vi "Generate Non Text Layer(s).vi"(0 "Library Path":path, 5 "new picture":picture, 11 "error in":errorcluster) -> (4 "Layers":refnum<class "Layer.lvclass">[](array[class]), 15 "error out":errorcluster)   [LabVIEW 2020, in "Text-Based VI Icon.lvlib"]
uses:
  <vilib>/LabVIEW Icon API/Set Text Icon/Text-Based VI Icon.lvlib
  <vilib>/LabVIEW Icon API/lv_icon/Classes/Layer/Layer.lvclass
  <vilib>/LabVIEW Icon API/lv_icon/Controls/Layer.ctl
  <vilib>/LabVIEW Icon API/Set Text Icon/User Visible Strings.vi
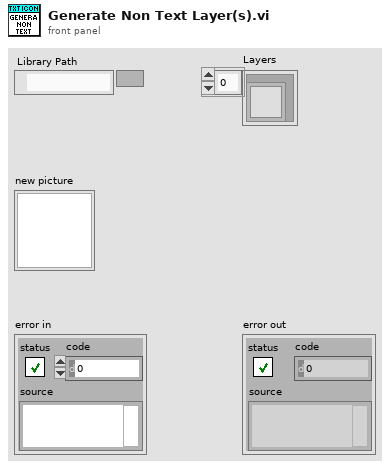
[diagram p1: front panel]
types:
  T1 = cluster{"left":i16, "top":i16, "right":i16, "bottom":i16}
  T2 = typedef "Layer.ctl" = cluster{"LayerIcon":picture, "LayerName":string, "Opacity":u8, "Visibility?":bool}
  T3 = typedef "imagedata.ctl" = cluster{"image type":i32, "image depth":i32, "image":u8[], "mask":u8[], "colors":u32[], "Rectangle":cluster{"left":i16, "top":i16, "right":i16, "bottom":i16}}
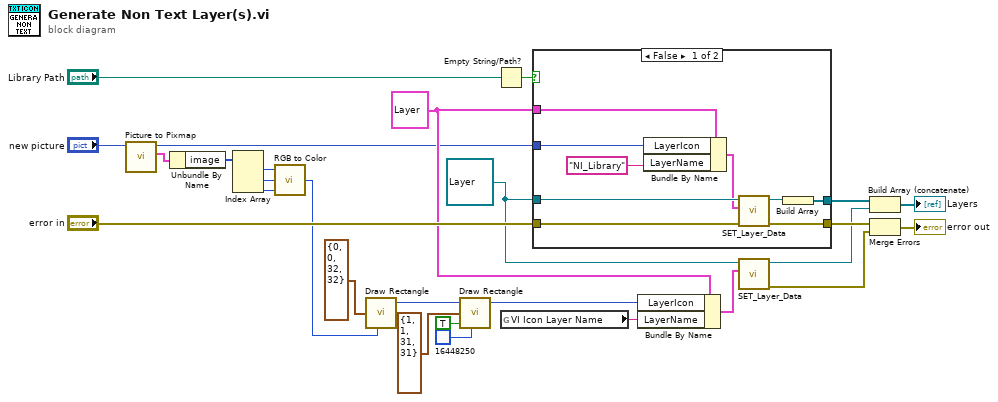
[diagram p0: block diagram]
diagram:
  w9 = T2 {"LayerIcon"=bytes[3102], "LayerName"="", "Opacity"=100, "Visibility?"=TRUE} ("Data")
  w25 = refnum<class "Layer.lvclass"> refnum ("Layer.lvclass in")
  n1 = call <vilib>:"Picture to Pixmap.vi"("picture"="new picture") -> ("image data"=w6:T3, "new picture"=w7:picture)  [unwired: 9 in]
  n2 = Unbundle By Name(w6) -> ("image"=w5:u8[])
  n3 = Index Array(array=w5) -> (element #1=w4:u8, element #2=w3:u8, element #3=w2:u8)  [unwired: 3 in]
  n4 = call <vilib>:"RGB to Color.vi"("B"=w2, "G"=w3, "R"=w4) -> ("Color"=w1:u32)
  n5 = call <vilib>:"Draw Rectangle.vi"("rect"=T1 {"left"=0, "top"=0, "right"=32, "bottom"=32}, "color(black)"=w1) -> ("new picture"=w23:picture)  [unwired: 7 in]
  n6 = call <vilib>:"Draw Rectangle.vi"("picture"=w23, "rect"=T1 {"left"=1, "top"=1, "right"=31, "bottom"=31}, "fill?(F)"=TRUE, "color(black)"=u32 16448250) -> ("new picture"=w21:picture)  [unwired: 5 in]
  n7 = Empty String/Path?(string/path="Library Path") -> (empty?=w26:bool)
  n8 = global read "User Visible Strings.vi" "VI Icon Layer Name"() -> (w17:string)
  n9 = case shown="False" w26 {
    tunnel: "error in" -> [w34 w37]
    tunnel: w25 -> [w36 _]
    tunnel: w9 -> [w35 _]
    tunnel: [w30 w37] -> w16
    tunnel: [w29 _] -> w14
    tunnel: w7 -> [w28 _]
    frame False {
      n10 = Bundle By Name(cluster=w35, "LayerIcon"=w28, "LayerName"="NI_Library") -> (w33:T2)
      n11 = call-dynamic "SET_Layer_Data.vi"("error in (no error)"=w34, "Data"=w33, "Layer.lvclass in"=w36) -> ("error out"=w30:errorcluster, "Layer.lvclass out"=w31:refnum<class "Layer.lvclass">)  [unwired: 7 in]
      n12 = Build Array(w31) -> (w29:refnum<class "Layer.lvclass">[])
    }
    frame True {
    }
  }
  n13 = Bundle By Name(cluster=w9, "LayerIcon"=w21, "LayerName"=w17) -> (w18:T2)
  n14 = call-dynamic "SET_Layer_Data.vi"("Data"=w18, "Layer.lvclass in"=w25) -> ("error out"=w15:errorcluster, "Layer.lvclass out"=w13:refnum<class "Layer.lvclass">)  [unwired: 8 in]
  n15 = Build Array (concatenate)(w14, w13) -> (→"Layers":refnum<class "Layer.lvclass">[])
  n16 = Merge Errors(w16, w15) -> (→"error out":errorcluster)
